vi "Mouse Down on Markers.vi"(8 "error in (no error)":errorcluster, 10 "Coords":T3, 11 "Refs":T1) -> (0 "error out":errorcluster, 1 "target axis":T2, 2 "Mouse down on axis marker?":bool, 3 "ScaleRef":refnum<vi>)   [LabVIEW 2021, in "RocketPlot.lvlib"]
uses:
  RocketPlot.lvlib
  <vilib>/Utility/miscctls.llb/LVPoint32TypeDef.ctl
  TypeDefs/Plot axis.ctl
  TypeDefs/Plot UI references.ctl
  Classes/RocketPlotHandle/RocketPlotHandle.lvclass
  <userlib>/bjustice/TipStripOOPanel/Classes/TipPanelHandle/TipPanelHandle.lvclass
  TypeDefs/Plot top row.ctl
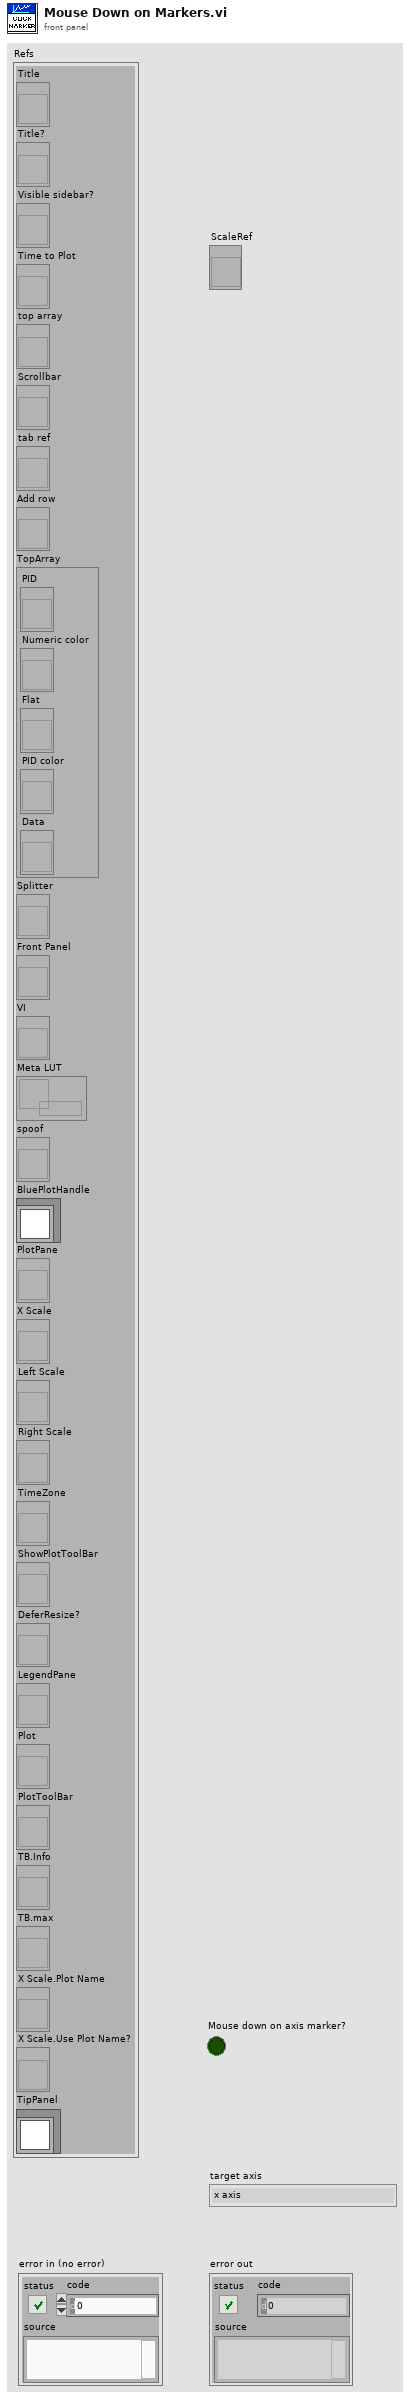
[diagram p1: front panel]
types:
  T1 = typedef "RocketPlot.lvlib/Plot UI references.ctl" = cluster{"Title":refnum<vi>, "Title?":refnum<vi>, "Visible sidebar?":refnum<vi>, "Time to Plot":refnum<vi>, "top array":refnum<vi>, "Scrollbar":refnum<vi>, "tab ref":refnum<vi>, "Add row":refnum<vi>, "TopArray":cluster{"PID":refnum<vi>, "Numeric color":refnum<vi>, "Flat":refnum<vi>, "PID color":refnum<vi>, "Data":refnum<vi>}, "Splitter":refnum<vi>, "Front Panel":refnum<vi>, "VI":refnum<vi>, "Meta LUT":refnum<data-value>, "spoof":refnum<vi>, "BluePlotHandle":refnum<class "RocketPlotHandle.lvclass">, "PlotPane":refnum<vi>, "X Scale":refnum<vi>, "Left Scale":refnum<vi>, "Right Scale":refnum<vi>, "TimeZone":refnum<vi>, "ShowPlotToolBar":refnum<vi>, "DeferResize?":refnum<vi>, "LegendPane":refnum<vi>, "Plot":refnum<vi>, "PlotToolBar":refnum<vi>, "TB.Info":refnum<vi>, "TB.max":refnum<vi>, "X Scale.Plot Name":refnum<vi>, "X Scale.Use Plot Name?":refnum<vi>, "TipPanel":refnum<class "TipPanelHandle.lvclass">}
  T2 = typedef "RocketPlot.lvlib/Plot axis.ctl" = enum16{"x axis", "left axis", "right axis"}
  T3 = typedef "LVPoint32TypeDef.ctl" = cluster{"Horizontal":i32, "Vertical":i32}
  T4 = typedef "LVRectTypeDef.ctl" = cluster{"Left":i16, "Top":i16, "Right":i16, "Bottom":i16}
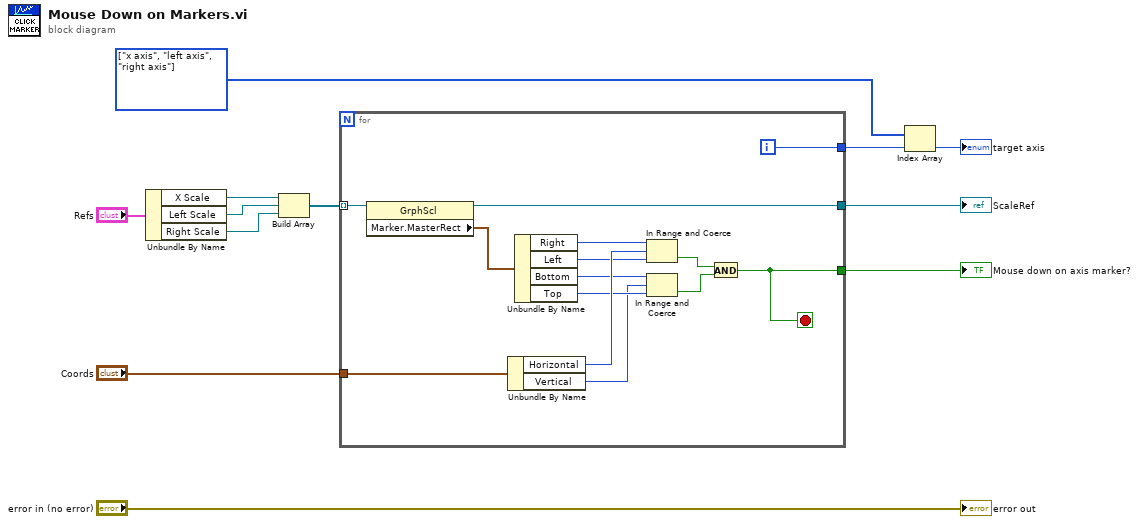
[diagram p0: block diagram]
diagram:
  w11 = T2[] [enum."x axis", enum."left axis", enum."right axis"] items=["x axis", "left axis", "right axis"] ("Array")
  n1 = Unbundle By Name("Refs") -> ("X Scale"=w9:refnum<vi>, "Left Scale"=w8:refnum<vi>, "Right Scale"=w7:refnum<vi>)
  n2 = Build Array(w9, w8, w7) -> (w6:refnum<vi>[])
  n3 = for {
    tunnel: "Coords" -> [w26]
    tunnel: [w17] -> w4
    tunnel: [w16] -> w12
    tunnel: w6 -> [w15] mode=indexing
    tunnel: [w13] -> w5
    i -> [w16]
    stop <- w17 stop-if-true
    n4 = property class="GrphScl"(reference=w15) -> (reference out=w13:refnum<vi>, "Marker.MasterRect"=w14:T4)  [unwired: 1 in, 1 out]
    n5 = Unbundle By Name(w26) -> ("Horizontal"=w25:i32, "Vertical"=w20:i32)
    n6 = Unbundle By Name(w14) -> ("Right"=w24:i16, "Left"=w23:i16, "Bottom"=w22:i16, "Top"=w21:i16)
    n7 = In Range and Coerce(upper limit=w24, x=w25, lower limit=w23) -> (In Range?=w19:bool)  [unwired: 1 out]
    n8 = In Range and Coerce(upper limit=w22, x=w20, lower limit=w21) -> (In Range?=w18:bool)  [unwired: 1 out]
    n9 = And(x=w19, y=w18) -> (x .and. y?=w17:bool)
  }
  "Mouse down on axis marker?" <- w4
  "ScaleRef" <- w5
  n10 = Index Array(array=w11, index=w12) -> (element=→"target axis":T2)
  "error out" <- "error in (no error)"
